vi "ReadPanesBounds.vi"(8 "error in (no error)":errorcluster, 11 "PentaPanesGUI in":refnum<class "PentaPanes.lvclass">) -> (0 "error out":errorcluster, 2 "Array":T1[](array[typedef]), 3 "PentaPanesGUI out":refnum<class "PentaPanes.lvclass">)   [LabVIEW 2022 SP3, in "PentaPanesLibrary.lvlib" / "PentaPanes.lvclass"]
uses:
  PentaPanes.lvclass
  <vilib>/Utility/miscctls.llb/LVBoundsTypeDef.ctl
  PentaPanes.lvclass/PentaPanes.ctl
panel:
  out "x-y":u32
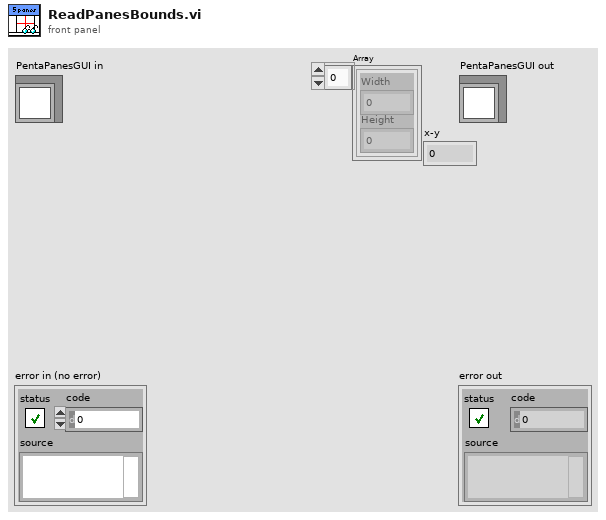
[diagram p1: front panel]
types:
  T1 = typedef "LVBoundsTypeDef.ctl" = cluster{"Width":i32, "Height":i32}
  T2 = typedef "PentaPanesLibrary.lvlib/PentaPanes.lvclass/PanesCluster.ctl" = cluster{"Top Pane":refnum<vi>, "Left Pane":refnum<vi>, "Center Pane":refnum<vi>, "Right Pane":refnum<vi>, "Bottom Pane":refnum<vi>}
  T3 = typedef "LVBoundsTypeDef.ctl" = cluster{"Width":u32, "Height":u32}
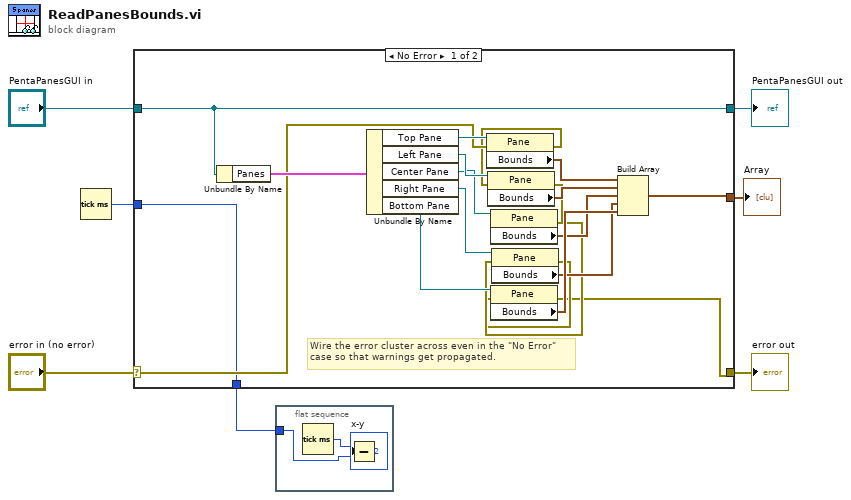
[diagram p0: block diagram]
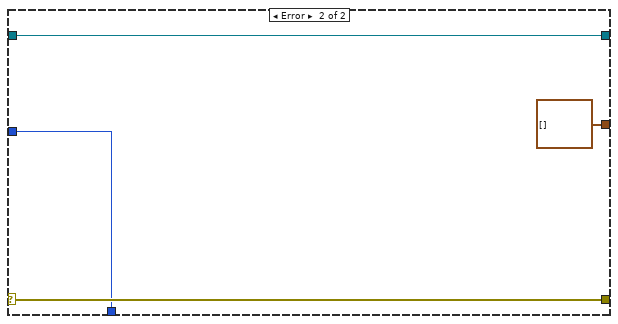
[diagram p2: hidden frame]
diagram:
  n1 = Tick Count (ms)() -> (millisecond timer value=w2:u32)
  n2 = case shown="No Error" "error in (no error)" {
    selector: "error in (no error)" -> [w14 w31]
    tunnel: [w9 w31] -> w6
    tunnel: [w27 w30] -> w4
    tunnel: "PentaPanesGUI in" -> [w27 w30]
    tunnel: [w15 T1[] []] -> w3
    tunnel: [w8 w28] -> w1
    tunnel: w2 -> [w8 w28]
    frame No Error {
      # "Wire the error cluster across even in the \"No Error\"\ncase so that warnings get propagated."
      n3 = Unbundle By Name(w27) -> ("Panes"=w26:T2)
      n4 = Unbundle By Name(w26) -> ("Top Pane"=w25:refnum<vi>, "Left Pane"=w24:refnum<vi>, "Center Pane"=w23:refnum<vi>, "Right Pane"=w22:refnum<vi>, "Bottom Pane"=w21:refnum<vi>)
      n5 = property class="Pane"(reference=w25, error in=w14) -> (error out=w13:errorcluster, "Bounds"=w16:T3)  [unwired: 1 out]
      n6 = property class="Pane"(reference=w24, error in=w13) -> (error out=w12:errorcluster, "Bounds"=w17:T3)  [unwired: 1 out]
      n7 = property class="Pane"(reference=w23, error in=w12) -> (error out=w11:errorcluster, "Bounds"=w18:T3)  [unwired: 1 out]
      n8 = property class="Pane"(reference=w22, error in=w11) -> (error out=w10:errorcluster, "Bounds"=w19:T3)  [unwired: 1 out]
      n9 = property class="Pane"(reference=w21, error in=w10) -> (error out=w9:errorcluster, "Bounds"=w20:T3)  [unwired: 1 out]
      n10 = Build Array(w16, w17, w18, w19, w20) -> (w15:T3[])
    }
    frame Error {
    }
  }
  "error out" <- w6
  "PentaPanesGUI out" <- w4
  "Array" <- w3
  n11 = flat-sequence {
    tunnel: w1 -> [w34]
    frame #0 {
      n12 = Tick Count (ms)() -> (millisecond timer value=w33:u32)
      n13 = Subtract(x=w33, y=w34) -> (x-y=→"x-y":u32)
    }
  }
